vi "Compile Script.vi"(0 "scripts manager in":refnum<class "scripts manager.lvclass">, 11 "error in (no error)":errorcluster) -> (4 "scripts manager out":refnum<class "scripts manager.lvclass">, 6 "compilation message":T1[](array[typedef]), 15 "error out":errorcluster)   [LabVIEW 2016, in "scripts manager.lvclass"]
uses:
  scripts manager.lvclass
  common/Validate_message.ctl
  scripts manager.lvclass/scripts manager.ctl
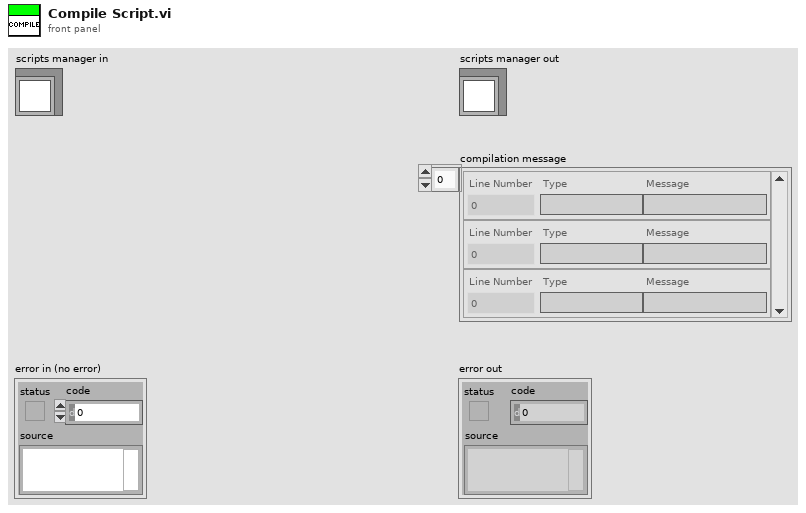
[diagram p1: front panel]
types:
  T1 = typedef "Validate_message.ctl" = cluster{"Line Number":i64, "Type":string, "Message":string}
  T2 = typedef "Line Details.ctl" = cluster{"Line#":i64, "Indent#":i64, "Function":string}
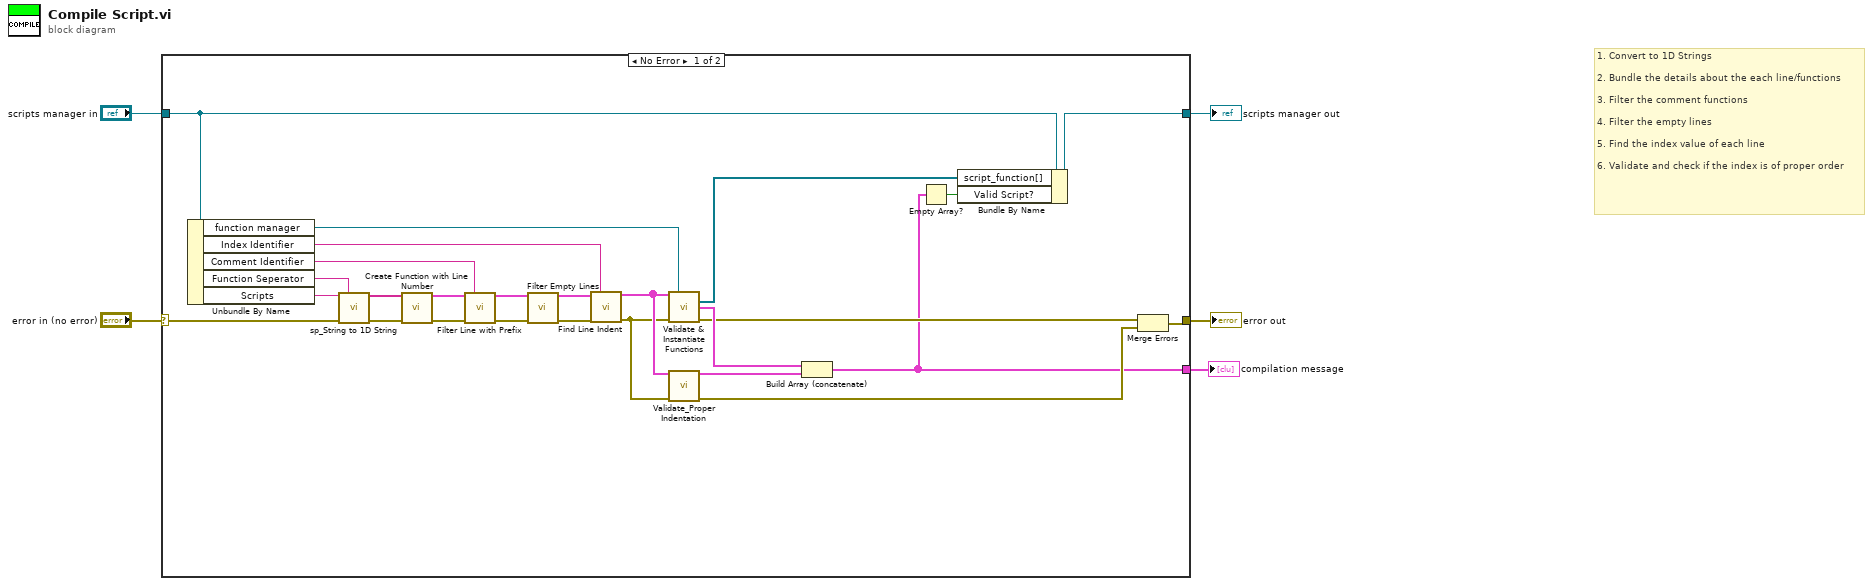
[diagram p0: block diagram]
diagram:
  # "1. Convert to 1D Strings\n\n2. Bundle the details about the each line/functions\n\n3. Filter the comment functions\n\n4. Filter the empty lines\n\n5. Find the index value of each line\n\n6. Validate and check if the index is of proper order"
  n1 = case shown="No Error" "error in (no error)" {
    selector: "error in (no error)" -> [w31 w33]
    tunnel: [w12 w33] -> w4
    tunnel: [w8 w32] -> w2
    tunnel: "scripts manager in" -> [w9 w32]
    tunnel: [w6 _] -> w1
    frame No Error {
      n2 = Unbundle By Name(w9) -> ("function manager"=w15:refnum<class "function manager.lvclass">, "Index Identifier"=w19:string, "Comment Identifier"=w24:string, "Function Seperator"=w29:string, "Scripts"=w30:string)
      n3 = call "sp_String to 1D String.vi"("script"=w30, "seperator"=w29, "error in (no error)"=w31) -> ("Script Lines"=w28:string[], "error out"=w27:errorcluster)  [unwired: 11 in]
      n4 = call "Create Function with Line Number.vi"("Script Lines in"=w28, "error in (no error)"=w27) -> ("Functions"=w25:T2[], "error out"=w26:errorcluster)  [unwired: 12 in]
      n5 = call "Filter Line with Prefix.vi"("Functions in"=w25, "Prefix"=w24, "error in (no error)"=w26) -> ("Functions"=w23:T2[], "error out"=w22:errorcluster)  [unwired: 11 in]
      n6 = call "Filter Empty Lines.vi"("Functions in"=w23, "error in (no error)"=w22) -> ("Functions"=w20:T2[], "error out"=w21:errorcluster)  [unwired: 12 in]
      n7 = call "Find Line Indent.vi"("Functions in"=w20, "Indent Identifier"=w19, "error in (no error)"=w21) -> ("Functions"=w17:T2[], "error out"=w16:errorcluster)  [unwired: 11 in]
      n8 = call "Validate & Instantiate Functions.vi"("Functions in"=w17, "function manager"=w15, "error in (no error)"=w16) -> ("Function [obj]"=w10:refnum<class "functionbase.lvclass">[], "Comiplation message"=w13:T1[], "error out"=w11:errorcluster)  [unwired: 9 in, 1 out]
      n9 = call "Validate_Proper Indentation.vi"("Functions in"=w17, "error in (no error)"=w16) -> ("Validation message"=w14:T1[], "error out"=w18:errorcluster)  [unwired: 12 in]
      n10 = Build Array (concatenate)(w13, w14) -> (w6:T1[])
      n11 = Empty Array?(array=w6) -> (empty?=w7:bool)
      n12 = Bundle By Name(cluster=w9, "script_function[]"=w10, "Valid Script?"=w7) -> (w8:refnum<class "scripts manager.lvclass">)
      n13 = Merge Errors(w11, w18) -> (w12:errorcluster)
    }
    frame Error {
    }
  }
  "error out" <- w4
  "scripts manager out" <- w2
  "compilation message" <- w1
